vi "BRig_dataExp_Cue2Switch_Count_First.vi"() -> (2 "output_Cue2Switch_Count_First":i32)   [LabVIEW 2014]
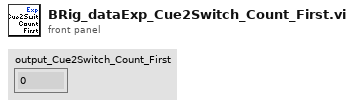
[diagram p1: front panel]
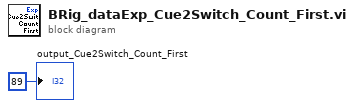
[diagram p0: block diagram]
diagram:
  "output_Cue2Switch_Count_First" <- 89 ("output_iBlock")
